vi "SplitChannels.vi"(10 "通道标尺":i32[](array[numeric]), 11 "所有通道数据":dbl[][](array[numeric])) -> (1 "反应性通道":dbl[][](array[numeric]), 2 "P2通道":dbl[][](array[numeric]), 3 "通量通道":dbl[][](array[numeric]))   [LabVIEW 2020]
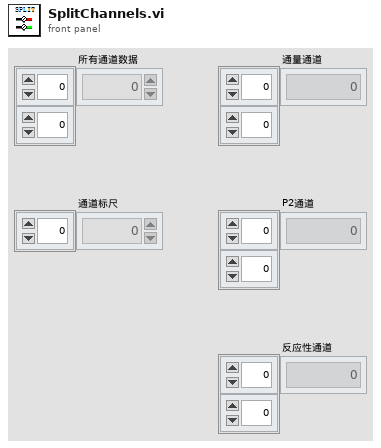
[diagram p1: front panel]
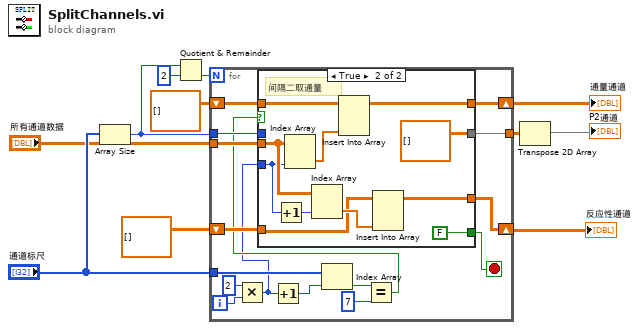
[diagram p0: block diagram]
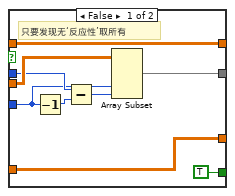
[diagram p2: hidden frame]
diagram:
  n1 = Array Size(array="通道标尺") -> (size(s)=w10:i32)
  n2 = Quotient & Remainder(x=w10, y=2) -> (floor(x/y)=w3:i32)  [unwired: 1 out]
  n3 = for {
    N: w3 -> [_]
    tunnel: "所有通道数据" -> [w25]
    tunnel: "通道标尺" -> [w16]
    shift-right: [w23] -> w5
    shift-left: dbl[][] [] ("type (empty)") -> [w24]
    tunnel: w10 -> [w20]
    tunnel: [w19] -> w4
    shift-right: [w17] -> w7
    shift-left: dbl[][] [] ("type (empty)") -> [w18]
    i -> [w27]
    stop <- w21 stop-if-true
    n4 = Multiply(x=2, y=w27) -> (x*y=w12:i32)
    n5 = Increment(x=w12) -> (x+1=w22:i32)
    n6 = Index Array(array=w16, index=w22) -> (element=w15:i32)
    n7 = Equal?(x=w15, y=7) -> (x = y?=w13:bool)
    n8 = case shown="True" w13 {
      tunnel: w25 -> [w34 w42]
      tunnel: w24 -> [w36 w47]
      tunnel: [w36 w45] -> w23
      tunnel: w12 -> [w30 w37]
      tunnel: [TRUE FALSE] -> w21
      tunnel: w20 -> [w33 _]
      tunnel: [w32 dbl[][] [] ("type (empty)")] -> w19
      tunnel: w18 -> [w31 w40]
      tunnel: [w31 w39] -> w17
      frame False {
        # "只要发现无‘反应性’取所有"
        n9 = Decrement(x=w30) -> (x-1=w28:i32)
        n10 = Subtract(x=w33, y=w28) -> (x-y=w29:i32)
        n11 = Array Subset(array=w34, index (col)=w30, length (col)=w29) -> (w32:dbl[][])  [unwired: 2 in]
      }
      frame True {
        # "间隔二取通量"
        n12 = Increment(x=w37) -> (x+1=w38:i32)
        n13 = Index Array(array=w42, index (col)=w37) -> (element=w46:dbl[])  [unwired: 1 in]
        n14 = Index Array(array=w42, index (col)=w38) -> (element=w41:dbl[])  [unwired: 1 in]
        n15 = Insert Into Array(array=w47, new element=w46) -> (w45:dbl[][])  [unwired: 2 in]
        n16 = Insert Into Array(array=w40, new element=w41) -> (w39:dbl[][])  [unwired: 2 in]
      }
    }
  }
  "反应性通道" <- w7
  "通量通道" <- w5
  n17 = Transpose 2D Array(2D array=w4) -> (transposed array=→"P2通道":dbl[][])
